vi "Read Signal Samples from File and Apply Filter.vi"() -> ()   [LabVIEW 2014]
uses:
  <vilib>/LabVIEW Universal Transcriptor/LabVIEW to Arduino Transcriptor/Transcriptors/System API/Serial println string.vi
  <vilib>/LabVIEW Universal Transcriptor/LabVIEW to Arduino Transcriptor/Transcriptors/System API/Serial print string.vi
  <vilib>/LabVIEW Universal Transcriptor/LabVIEW Universal Transcriptor SD Card Library/File.lvclass
  <vilib>/LabVIEW Universal Transcriptor/LabVIEW Universal Transcriptor SD Card Library/LabVIEW Universal Transcriptor SD Card Library.lvlib
  <vilib>/LabVIEW Universal Transcriptor/LabVIEW to Arduino Transcriptor/Transcriptors/System API/System Serial Library Variables/System Serial Library Variables.lvlib
panel:
  out "String Buffer":string
  out "error out":errorcluster
  in  "Error In":errorcluster
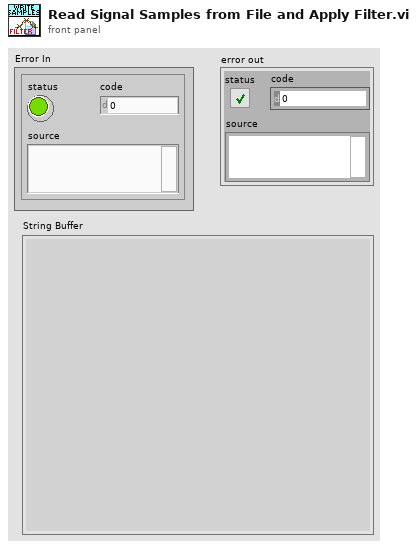
[diagram p1: front panel]
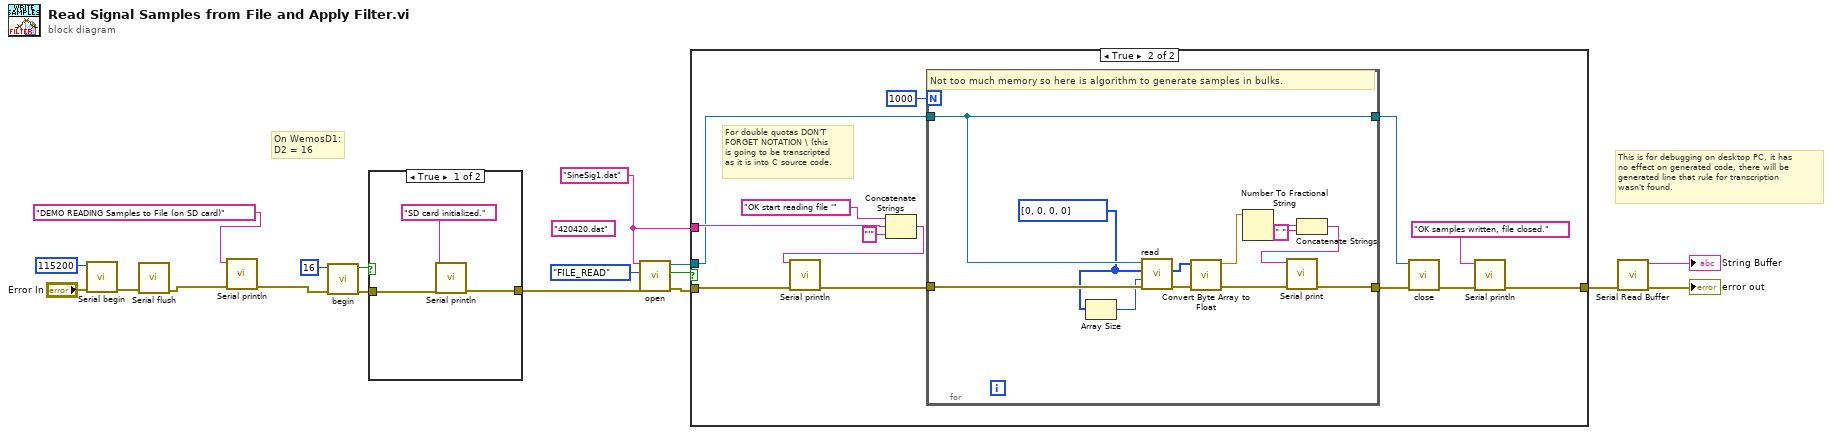
[diagram p0: block diagram]
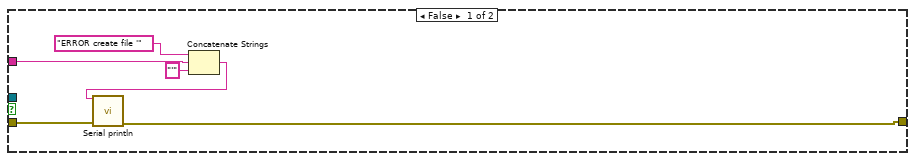
[diagram p2: hidden frame]
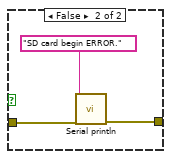
[diagram p3: hidden frame]
diagram:
  w1 = "SineSig1.dat" ("filepath")
  (unwired) "420420.dat" ("filepath")
  # "On WemosD1:\nD2 = 16"
  # "This is for debugging on desktop PC, it has\nno effect on generated code, there will be\ngenerated line that rule for transcription\nwasn't found."
  n1 = call <vilib>:"Serial begin.vi"("Error In"="Error In", "speed (Bd)"=115200) -> ("Error Out"=w18:errorcluster)  [unwired: 9 in]
  n2 = call <vilib>:"Serial flush.vi"("Error In"=w18) -> ("Error Out"=w16:errorcluster)  [unwired: 10 in]
  n3 = call-poly <vilib>:"Serial println.vi"("Error In"=w16, "string in"="DEMO READING Samples to File (on SD card)") -> ("Error Out"=w14:errorcluster)  [unwired: 9 in]
  n4 = call <vilib>:"begin.vi"("Error In"=w14, "CS pin (optional)"=u8 16) -> ("Error Out"=w11:errorcluster, "success?"=w12:bool)  [unwired: 8 in]
  n5 = case shown="True" w12 {
    tunnel: w11 -> [w21 w24]
    tunnel: [w19 w22] -> w2
    frame True {
      n6 = call-poly <vilib>:"Serial println.vi"("Error In"=w21, "string in"="SD card initialized.") -> ("Error Out"=w19:errorcluster)  [unwired: 9 in]
    }
    frame False {
      n7 = call-poly <vilib>:"Serial println.vi"("Error In"=w24, "string in"="SD card begin ERROR.") -> ("Error Out"=w22:errorcluster)  [unwired: 9 in]
    }
  }
  n8 = call <vilib>:"open.vi"("Error In"=w2, "mode"=enum16{"FILE_READ", "FILE_WRITE"}."FILE_READ", "filepath"=w1) -> ("Error Out"=w9:errorcluster, "opened?"=w8:bool, "File out"=w7:refnum<class "File.lvclass">)  [unwired: 6 in]
  n9 = case shown="True" w8 {
    tunnel: w9 -> [w26 w40]
    tunnel: w1 -> [w30 w39]
    tunnel: [w25 w32] -> w6
    tunnel: w7 -> [_ w37]
    frame False {
      n10 = Concatenate Strings("ERROR create file '" ("string in"), w30, "'" ("string")) -> (w27:string)
      n11 = call-poly <vilib>:"Serial println.vi"("Error In"=w26, "string in"=w27) -> ("Error Out"=w25:errorcluster)  [unwired: 9 in]
    }
    frame True {
      # "For double quotas DON'T\nFORGET NOTATION \\ (this\nis going to be transcripted\nas it is into C source code."
      n12 = Concatenate Strings("OK start reading file '" ("string in"), w39, "'" ("string")) -> (w41:string)
      n13 = call-poly <vilib>:"Serial println.vi"("Error In"=w40, "string in"=w41) -> ("Error Out"=w38:errorcluster)  [unwired: 9 in]
      n14 = for {
        N: 1000 -> [_]
        tunnel: w38 -> [w51]
        tunnel: w37 -> [w50]
        tunnel: [w50] -> w36
        tunnel: [w55] -> w31
        w49 = u8[] [0, 0, 0, 0] ("buffer")
        # "Not too much memory so here is algorithm to generate samples in bulks."
        n15 = Array Size(array=w49) -> (size(s)=w48:i32)
        n16 = call-dynamic "read.vi"("error in (no error)"=w51, "length"=w48, "buffer"=w49, "File in"=w50) -> ("error out"=w46:errorcluster, "buffer out"=w47:u8[])  [unwired: 6 in]
        n17 = call "Convert Byte Array to Float.vi"("error in"=w46, "buffer in"=w47) -> ("error out"=w45:errorcluster, "number out"=w44:sgl)  [unwired: 8 in]
        n18 = Number To Fractional String(number=w44) -> (F-format string=w53:string)  [unwired: 3 in]
        n19 = Concatenate Strings(w53, " " ("element")) -> (w52:string)
        n20 = call-poly <vilib>:"Serial print.vi"("Error In"=w45, "string in"=w52) -> ("Error Out"=w55:errorcluster)  [unwired: 9 in]
      }
      n21 = call-dynamic "close.vi"("error in (no error)"=w31, "File in"=w36) -> ("error out"=w33:errorcluster)  [unwired: 9 in]
      n22 = call-poly <vilib>:"Serial println.vi"("Error In"=w33, "string in"="OK samples written, file closed.") -> ("Error Out"=w32:errorcluster)  [unwired: 9 in]
    }
  }
  n23 = call <vilib>:"Serial Read Buffer.vi"("Error In"=w6) -> ("Error Out"=→"error out":errorcluster, "String Buffer"=→"String Buffer":string)  [unwired: 9 in]
